vi "Read EntryTick.vi"(8 "error in (no error)":errorcluster, 11 "ReceiverState in":refnum<class "ConnectCommand.lvclass">) -> (0 "error out":errorcluster, 2 "TimeInState":u32, 3 "ReceiverState out":refnum<class "ConnectCommand.lvclass">)   [LabVIEW 2013]
uses:
  Connect Command/ConnectCommand.lvclass
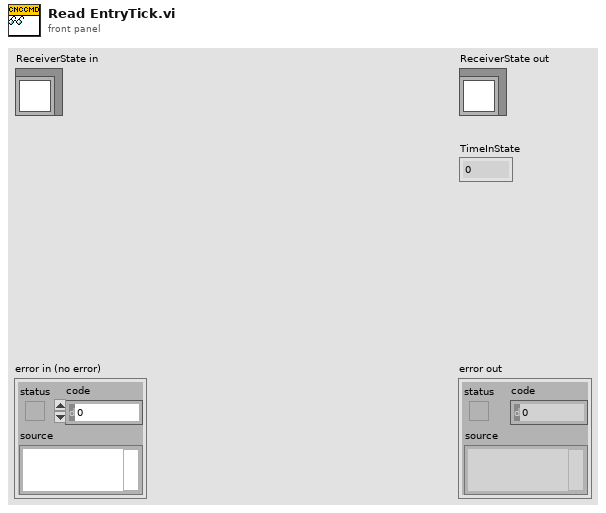
[diagram p1: front panel]
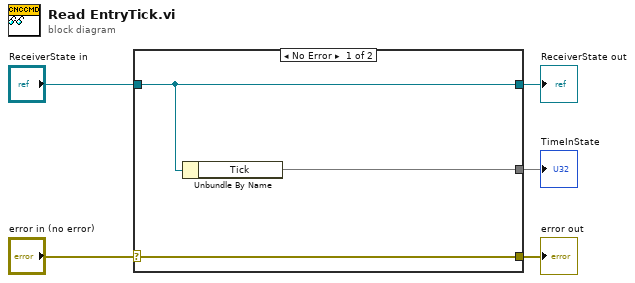
[diagram p0: block diagram]
diagram:
  n1 = case shown="No Error" "error in (no error)" {
    selector: "error in (no error)" -> [w8 w9]
    tunnel: [w8 w9] -> w4
    tunnel: [w7 w10] -> w2
    tunnel: "ReceiverState in" -> [w7 w10]
    tunnel: [w6 _] -> w1
    frame No Error {
      n2 = Unbundle By Name(w7) -> ("Tick"=w6)
    }
    frame Error {
    }
  }
  "error out" <- w4
  "ReceiverState out" <- w2
  "TimeInState" <- w1
